vi "FanModelInter.vi"(6 "DirVecs":dbl[][](array[numeric]), 8 "Length":dbl, 9 "Point":dbl[](array[numeric]), 11 "TriangleInfo":T1) -> (2 "TriangleIndexes":i32[](array[numeric]), 3 "Dists":cluster{dbl[]}[](array[cluster]))   [LabVIEW 2014]
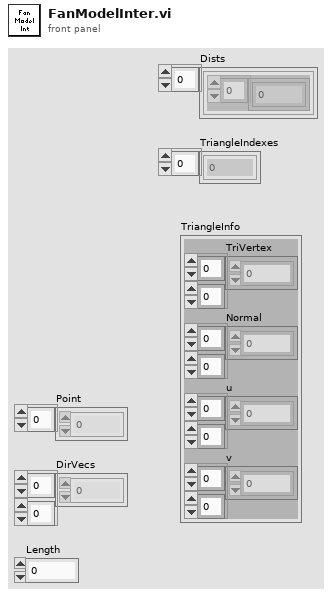
[diagram p1: front panel]
types:
  T1 = cluster{"TriVertex":dbl[][], "Normal":dbl[][], "u":dbl[][], "v":dbl[][]}
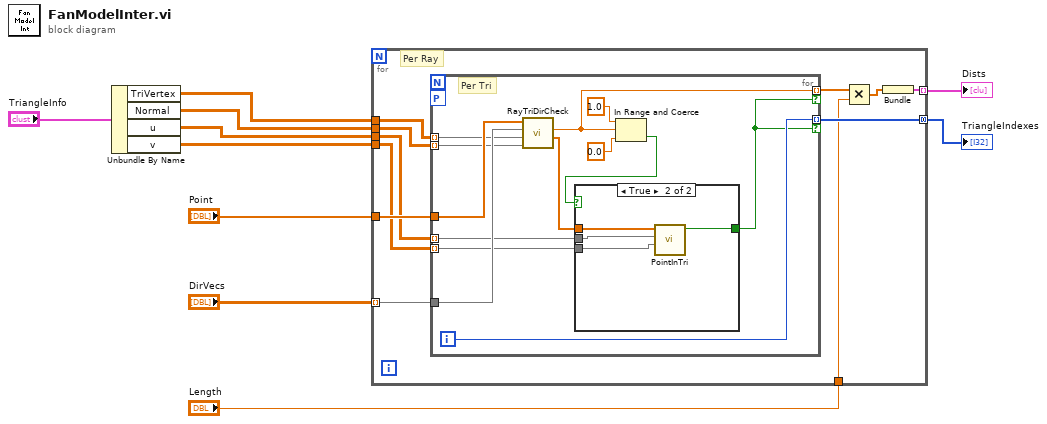
[diagram p0: block diagram]
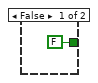
[diagram p2: hidden frame]
diagram:
  n1 = Unbundle By Name("TriangleInfo") -> ("TriVertex"=w4:dbl[][], "Normal"=w3:dbl[][], "u"=w2:dbl[][], "v"=w1:dbl[][])
  n2 = for {
    tunnel: w4 -> [w19]
    tunnel: w3 -> [w18]
    tunnel: w2 -> [w17]
    tunnel: w1 -> [w16]
    tunnel: "Point" -> [w21]
    tunnel: "DirVecs" -> [w20] mode=indexing
    tunnel: [w14] -> w9 mode=indexing
    tunnel: [w15] -> w8 mode=concatenating
    tunnel: "Length" -> [w12]
    # "Per Ray"
    n3 = for {
      tunnel: w21 -> [w34]
      tunnel: w20 -> [w33]
      tunnel: w19 -> [w32] mode=indexing
      tunnel: w18 -> [w31] mode=indexing
      tunnel: w17 -> [w26] mode=indexing
      tunnel: w16 -> [w25] mode=indexing
      tunnel: [w24] -> w13 mode=indexing if=w22
      tunnel: [w23] -> w15 mode=indexing if=w22
      workers-P: _ -> [_]
      i -> [w23]
      # "Per Tri"
      n4 = call "RayTriDirCheck.vi"("Normal"=w31, "TriVertex"=w32, "Dir"=w33, "P0"=w34) -> ("w"=w27:dbl[], "r"=w24:dbl)  [unwired: 5 in, 1 out]
      n5 = In Range and Coerce(upper limit=1.0, x=w24, lower limit=0.0) -> (In Range?=w28:bool)  [unwired: 1 out]
      n6 = case shown="True" w28 {
        tunnel: w27 -> [_ w39]
        tunnel: w26 -> [_ w38]
        tunnel: w25 -> [_ w37]
        tunnel: [FALSE ("PointInTri") w36] -> w22
        frame False {
        }
        frame True {
          n7 = call "PointInTri.vi"("v"=w37, "u"=w38, "w"=w39) -> ("PointInTri"=w36:bool)  [unwired: 8 in]
        }
      }
    }
    n8 = Multiply(x=w13, y=w12) -> (x*y=w11:dbl[])
    n9 = Bundle(w11) -> (w14:cluster{dbl[]})  [unwired: 1 in]
  }
  "Dists" <- w9
  "TriangleIndexes" <- w8
